vi "linear curve fitting.vi"() -> ()   [LabVIEW 2018]
uses:
  <vilib>/Utility/file.llb/Read Delimited Spreadsheet (DBL).vi
  <vilib>/Analysis/NI_AALPro.lvlib
panel:
  out "Prepared by \nthe project":string
  out "Linear Curve Fitting":dbl[](graph)
  out "Data":dbl[][](array[numeric])
  in  "Measurement file \nwith extension Txt":path
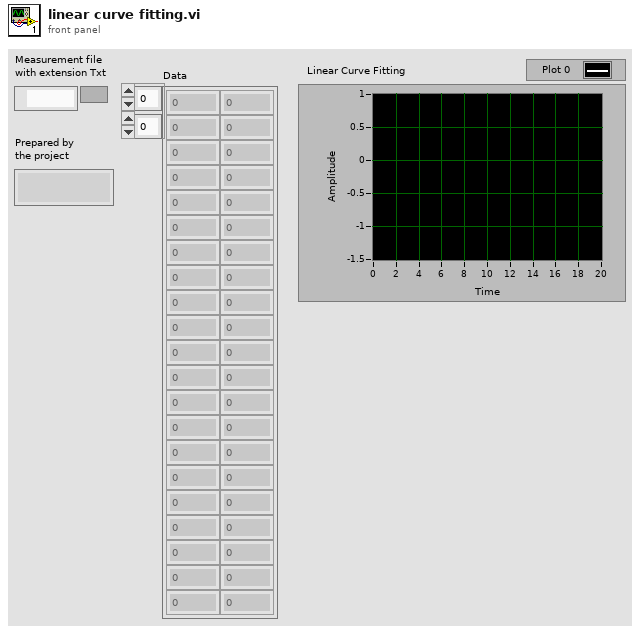
[diagram p1: front panel]
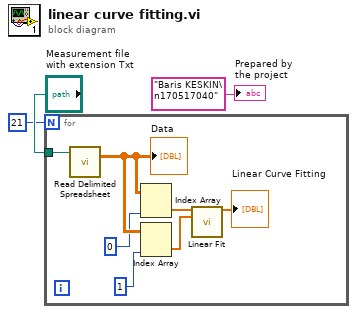
[diagram p0: block diagram]
diagram:
  n1 = for {
    N: 21 -> [_]
    tunnel: "Measurement file \nwith extension Txt" -> [w10]
    n2 = call-poly <vilib>:"Read Delimited Spreadsheet.vi"("file path (dialog if empty)"=w10) -> ("all rows"=w9:dbl[][])  [unwired: 9 in, 5 out]
    "Data" <- w9
    n3 = Index Array(array=w9, index (col)=0 ("disabled index (col)")) -> (element=w6:dbl[])  [unwired: 1 in]
    n4 = Index Array(array=w9, index (col)=1 ("disabled index (col)")) -> (element=w5:dbl[])  [unwired: 1 in]
    n5 = call <vilib>:"Linear Fit.vi"("Y"=w6, "X"=w5) -> ("Best Linear Fit"=→"Linear Curve Fitting":dbl[])  [unwired: 9 in, 4 out]
  }
  "Prepared by \nthe project" <- "Baris KESKIN\n170517040"
